vi "iPad Control Experimenting.vi"() -> ()   [LabVIEW 2014]
uses:
  controls/UI DataSam.ctl
  globals/UI Network Stream EndpointsSam.vi
panel:
  in  "Controller Address":string="172.16.0.1"
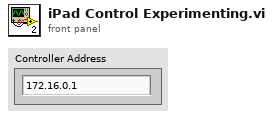
[diagram p1: front panel]
types:
  T1 = typedef "UI DataSam.ctl" = cluster{"Message":string, "Data":variant}
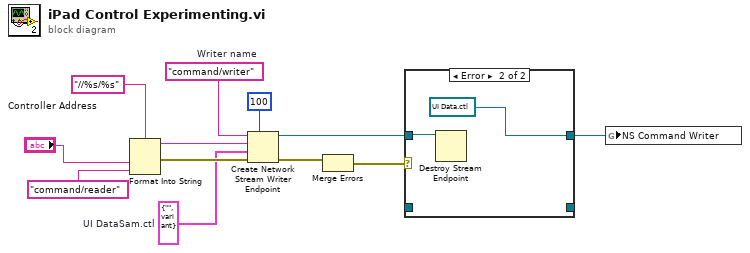
[diagram p0: block diagram]
diagram:
  w1 = T1 {"Message"="", "Data"=variant}  # UI DataSam.ctl
  w7 = "command/writer"  # Writer name
  n1 = Format Into String(format string="//%s/%s", "Controller Address", "command/reader" ("input 2")) -> (resulting string=w9:string, error out=w10:errorcluster)  [unwired: 2 in]
  n2 = Create Network Stream Writer Endpoint(7:100 ("writer buffer size"), 8:w10, 9:w1, 10:w9, 11:w7) -> (0:w5:errorcluster, 3:w6:refnum<k21>)  [unwired: 2 in]
  n3 = Merge Errors(w5) -> (w4:errorcluster)  [unwired: 1 in]
  n4 = case shown="Error" w4 {
    tunnel: w6 -> [w14 w16]
    tunnel: [w14 refnum<k21> refnum ("Writer name")] -> w2
    tunnel: [w13 _] -> _
    tunnel: _ -> [w13 _]
    frame No Error {
    }
    frame Error {
      n5 = Destroy Stream Endpoint(11:w16) -> ()  [unwired: 1 in, 1 out]
    }
  }
  n6 = global write "UI Network Stream EndpointsSam.vi" "NS Command Writer"(w2) -> ()
